vi "PH_Numbers.Set Precision of Number II.vi"(0 "Number":dbl format="%#_12g", 1 "Precision (6)":u8=6) -> (2 "Precision":i32)   [LabVIEW 2014, in "PH_Common.lvlib"]
doc: "This VI is forseen for proper translation of a double to a string: It kicks out the last zeros after the decimal point up to the wired input \"precision\"."
uses:
  PH_Common.lvlib
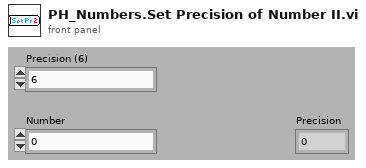
[diagram p1: front panel]
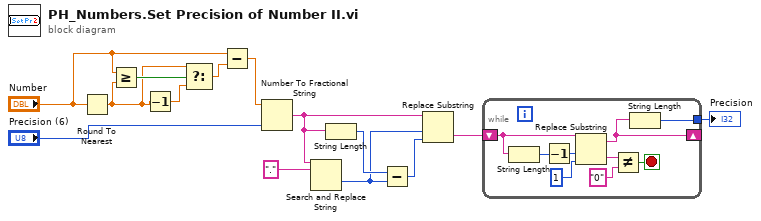
[diagram p0: block diagram]
diagram:
  n1 = Round To Nearest(number="Number") -> (nearest integer value=w5:dbl)
  n2 = Greater Or Equal?(x="Number", y=w5) -> (x >= y?=w6:bool)
  n3 = Decrement(x=w5) -> (x-1=w4:dbl)
  n4 = Select(t=w5, s=w6, f=w4) -> (s? t:f=w3:dbl)
  n5 = Subtract(x="Number", y=w3) -> (x-y=w1:dbl)
  n6 = Number To Fractional String(number=w1, precision (6)="Precision (6)") -> (F-format string=w10:string)  [unwired: 2 in]
  n7 = Search and Replace String(input string=w10, search string="." ("regular expression")) -> (offset past replacement=w8:i32)  [unwired: 6 in, 3 out]
  n8 = String Length(string=w10) -> (length=w9:i32)
  n9 = Subtract(x=w9, y=w8) -> (x-y=w7:i32)
  n10 = Replace Substring(2:w7, 3:w8, 5:w10) -> (0:w11:string)  [unwired: 1 in, 1 out]
  n11 = while {
    shift-right: [w17] -> _
    shift-left: w11 -> [w23]
    tunnel: [w16] -> w13
    stop <- w15 stop-if-true
    n12 = String Length(string=w23) -> (length=w22:i32)
    n13 = Decrement(x=w22) -> (x-1=w21:i32)
    n14 = Replace Substring(2:1 ("length (len. of substring)"), 3:w21, 5:w23) -> (0:w19:string, 1:w17:string)  [unwired: 1 in]
    n15 = Not Equal?(x=w19, y="0") -> (x != y?=w15:bool)
    n16 = String Length(string=w17) -> (length=w16:i32)
  }
  "Precision" <- w13
